vi "Actor Core.vi"(8 "error in":errorcluster, 11 "MediatorBusMonitor In":refnum<class "MediatorBusMonitor.lvclass">) -> (0 "error out":errorcluster, 3 "Actor out":refnum<class "Actor.lvclass">)   [LabVIEW 2015, in "Mediator.lvlib" / "MediatorBusMonitor.lvclass"]
doc: "(<B>Filename</B>: Actor Framework.lvlib:Actor.lvclass:Actor Core.vi)\n\nReceives messages to the actor, reacts to them, and initiates any error handling that may shut the actor down.\n\nDescendant classes may override this VI to append parallel tasks for the actor to complete while it handles messages. Overrides use the Call Parent Method node.\n\n<License>\nCopyright © 2017 Composed Systems, LLC | All rights reserved\nwww.composed.io\n\nAuthor: Ethan Stern <ethan.stern@composed.io>\n\nThis software is provided \"AS IS\" WITHOUT WARRANTIES, either express or implied, AND IS FOR EDUCATIONAL PURPOSES ONLY.\n</License>"
uses:
  MediatorBusMonitor.lvclass
  <vilib>/ActorFramework/Actor/Actor.lvclass
  MediatorBusMonitor.lvclass/MediatorBusMonitor.ctl
  <vilib>/ActorFramework/Actor/Actor.lvclass/Actor.ctl
  <vilib>/ActorFramework/Message Enqueuer/Message Enqueuer.lvclass/Message Enqueuer.ctl
  AutoRegistration/ActorAutoRegistration/ActorAutoRegistration.lvclass/ActorAutoRegistration.ctl
  <vilib>/ActorFramework/Message Enqueuer/Init from Existing Queue.vi
  AutoRegistration/AutoRegistration/Register for Panel Events.vi
  IMediator/IMediatorBusMonitor/MediatorBusMonitor/IMediatorBusMonitor.lvclass
  <vilib>/ActorFramework/Message Enqueuer/Message Enqueuer.lvclass
  AutoRegistration/ActorAutoRegistration/ActorAutoRegistration.lvclass
panel:
  in  "Multicolumn Listbox":i32(listbox)
  in  "Update Period":dbl=1.0 min=0.0 max=60.0 step=0.001 format="%#.3g sec"
  in  "Clear History":bool
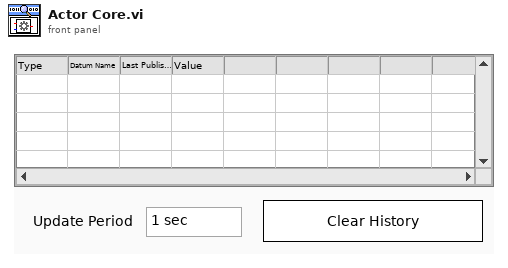
[diagram p1: front panel]
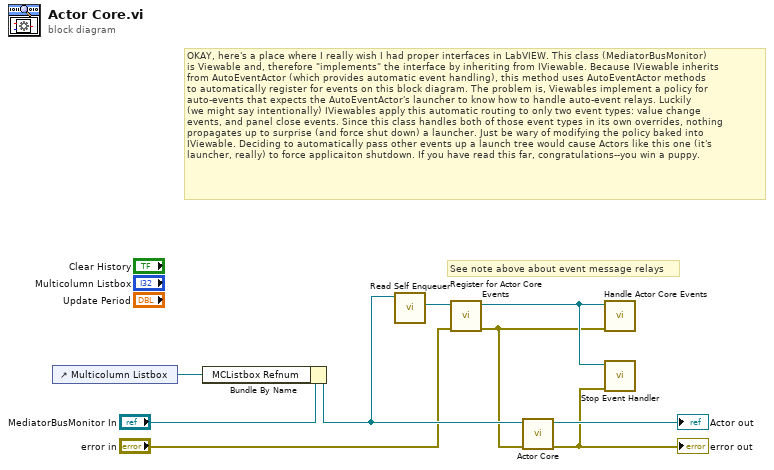
[diagram p0: block diagram]
diagram:
  # "See note above about event message relays"
  # "OKAY, here's a place where I really wish I had proper interfaces in LabVIEW. This class (MediatorBusMonitor)\nis Viewable and, therefore \"implements\" the interface by inheriting from IViewable. Because IViewable inherits\nfrom AutoEventActor (which provides automatic event handling), this method uses AutoEventActor methods\nto automatically register for events on this block diagram. The problem is, Viewables implement a policy for\nauto-events that expects the AutoEventActor's launcher to know how to handle auto-event relays. Luckily\n(we might say intentionally) IViewables apply this automatic routing to only two event types: value change\nevents, and panel close events. Since this class handles both of those event types in its own overrides, nothing\npropagates up to surprise (and force shut down) a launcher. Just be wary of modifying the policy baked into\nIViewable. Deciding to automatically pass other events up a launch tree would cause Actors like this one (it's\nlauncher, really) to force applicaiton shutdown. If you have read this far, congratulations--you win a puppy."
  n1 = control-ref of="Multicolumn Listbox"() -> (w7:refnum<vi>)
  n2 = Bundle By Name(cluster="MediatorBusMonitor In", "MCListbox Refnum"=w7) -> (w6:refnum<class "MediatorBusMonitor.lvclass">)
  n3 = call <vilib>:"Read Self Enqueuer.vi"("Actor"=w6) -> ("Self Enqueuer"=w3:refnum<class "Message Enqueuer.lvclass">)  [unwired: 10 in]
  n4 = call "Register for Actor Core Events.vi"("error in (no error)"="error in", "Actor Enqueuer"=w3) -> ("error out"=w1:errorcluster, "ActorAutoRegistration Out"=w5:refnum<class "ActorAutoRegistration.lvclass">)  [unwired: 8 in]
  n5 = call-parent "Actor Core.vi"("error in"=w1, "IViewable In"=w6) -> ("error out"=w4:errorcluster, "Actor out"=→"Actor out":refnum<class "Actor.lvclass">)  [unwired: 8 in]
  "error out" <- w4
  n6 = call-dynamic "Handle Actor Core Events.vi"("error in (no error)"=w1, "ActorAutoRegistration"=w5) -> ()  [unwired: 9 in, 1 out]
  n7 = call-dynamic "Stop Event Handler.vi"("error in (no error)"=w4, "ActorAutoRegistration In"=w5) -> ()  [unwired: 9 in, 1 out]
